vi "standard deviationsubvi.vi"(10 "array 2":dbl[](array[numeric]), 11 "array":dbl[](array[numeric])) -> (3 "Numeric":dbl)   [LabVIEW 2013]
panel:
  in  "array 4":dbl[](array[numeric])
  in  "array 3":dbl[](array[numeric])
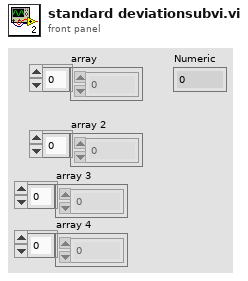
[diagram p1: front panel]
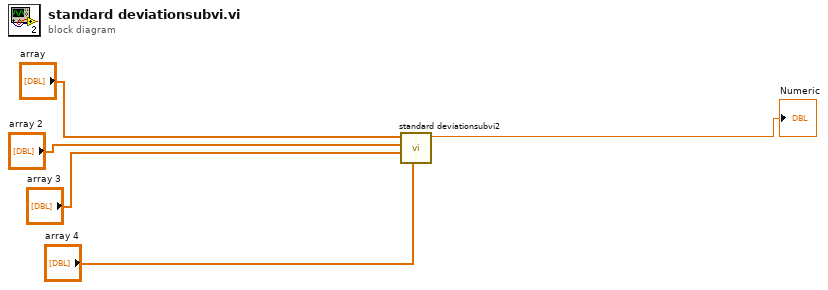
[diagram p0: block diagram]
diagram:
  n1 = call "standard deviationsubvi2.vi"("array 4"="array 4", "array 3"="array 3", "array 2"="array 2", "array"="array") -> ("Numeric"=→"Numeric":dbl)  [unwired: 7 in]
